vi "make_cursor_text.vi"(4 "Track Eye":T3, 5 "Cursor Position":T4, 6 "Scale":T1, 7 "Cursor Text":T2={"Cursor Name"="Cursor0", "Font Size"=7, "Show Position"=TRUE, "Show Name"=TRUE, "Text Color"=0, "Back Color"=16754450, "Opacity"=0.5}, 9 "Point Size":dbl, 10 "Cursor Name":string, 11 "Scene Cursor Object In":refnum<vi>) -> (3 "Scene Cursor Object Out":refnum<vi>)   [LabVIEW 2020, in "3DPC_SurfacePlot.xctl"]
uses:
  <vilib>/Native 3D Graph/xcontrol/3DPC_SurfacePlot.xctl
  <vilib>/Native 3D Graph/typedefs/prop_cursor_position.ctl
  <vilib>/Native 3D Graph/typedefs/track_eye.ctl
  <vilib>/Native 3D Graph/typedefs/vector.ctl
  <vilib>/Native 3D Graph/typedefs/prop_cursor_text.ctl
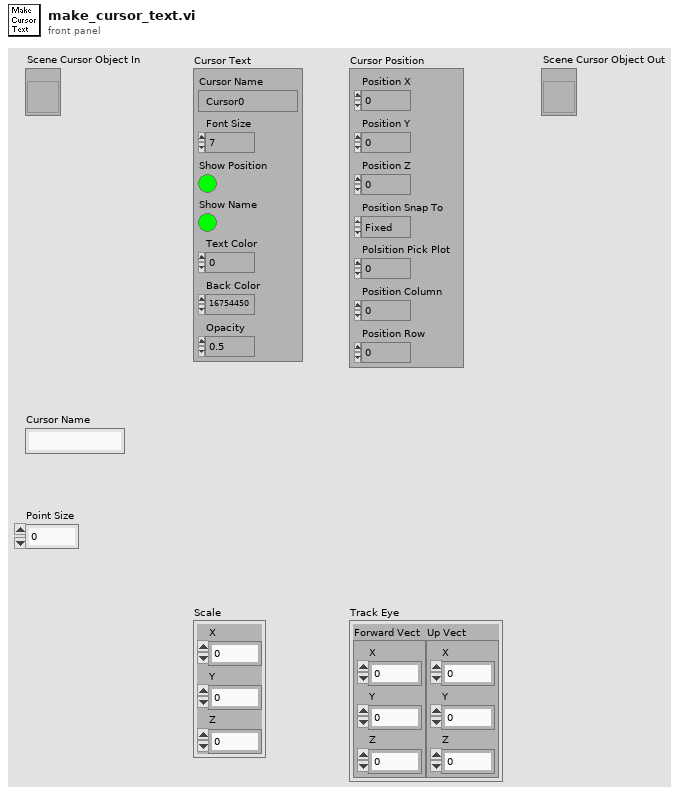
[diagram p1: front panel]
types:
  T1 = typedef "3DPC_SurfacePlot.xctl/vector.ctl" = cluster{"X":sgl, "Y":sgl, "Z":sgl}
  T2 = typedef "3DPC_SurfacePlot.xctl/prop_cursor_text.ctl" = cluster{"Cursor Name":string, "Font Size":i32, "Show Position":bool, "Show Name":bool, "Text Color":u32, "Back Color":u32, "Opacity":dbl}
  T3 = typedef "3DPC_SurfacePlot.xctl/track_eye.ctl" = cluster{"Forward Vect":T1, "Up Vect":T1}
  T4 = typedef "3DPC_SurfacePlot.xctl/prop_cursor_position.ctl" = cluster{"Position X":dbl, "Position Y":dbl, "Position Z":dbl, "Position Snap To":enum16{"Fixed", "Nearest Plot", "Snap to Plot"}, "Polsition Pick Plot":u16, "Position Column":i32, "Position Row":i32}
  T5 = enum8{"X-Y", "Y-Z", "X-Z", "Reversed X-Y", "Reversed Y-Z", "Reversed X-Z", "Screen"}
  T6 = enum16{"Normal Bin", "Opaque Bin", "Transparent Bin"}
  T7 = cluster{"Position X":dbl, "Position Y":dbl, "Position Z":dbl}
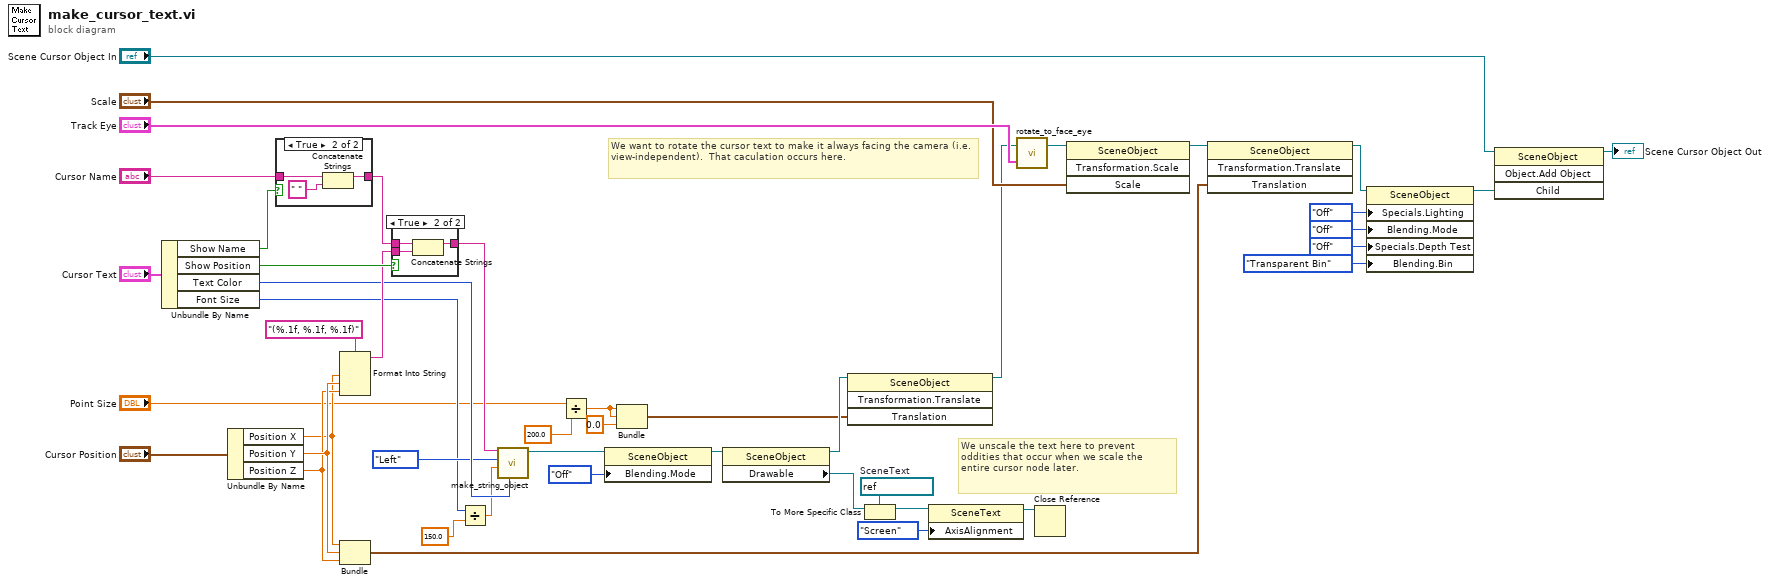
[diagram p0: block diagram]
diagram:
  w20 = refnum<vi> refnum  # SceneText
  # "We unscale the text here to prevent oddities that occur when we scale the entire cursor node later."
  # "We want to rotate the cursor text to make it always facing the camera (i.e. view-independent).  That caculation occurs here."
  n1 = Unbundle By Name("Cursor Text") -> ("Show Name"=w34:bool, "Show Position"=w33:bool, "Text Color"=w29:u32, "Font Size"=w12:i32)
  n2 = Unbundle By Name("Cursor Position") -> ("Position X"=w8:dbl, "Position Y"=w44:dbl, "Position Z"=w28:dbl)
  n3 = case shown="True" w34 {
    tunnel: "Cursor Name" -> [_ w48]
    tunnel: [_ w46] -> w32
    frame False {
    }
    frame True {
      n4 = Concatenate Strings(w48, " " ("string")) -> (w46:string)
    }
  }
  n5 = Format Into String(format string="(%.1f, %.1f, %.1f)", w8, w44, w28) -> (resulting string=w31:string)  [unwired: 2 in, 1 out]
  n6 = Bundle("Position X"=w8, "Position Y"=w44, "Position Z"=w28) -> (w42:T7)  [unwired: 1 out]
  n7 = case shown="True" w33 {
    tunnel: w32 -> [w49 w52]
    tunnel: w31 -> [_ w51]
    tunnel: [w49 w50] -> w30
    frame False {
    }
    frame True {
      n8 = Concatenate Strings(w52, w51) -> (w50:string)
    }
  }
  n9 = Divide(x=w12, y=150.0) -> (x/y=w9:dbl)
  n10 = call <vilib>:"make_string_object.vi"("Color"=w29, "Font Size"=w9, "Alignment:Horizontal"=enum8{"Left", "Right", "Center"}."Left", "String"=w30) -> ("String Object Out"=w26:refnum<vi>)  [unwired: 7 out]
  n11 = Divide(x="Point Size", y=200.0) -> (x/y=w3:dbl)
  n12 = property class="SceneObject"(reference=w26, "Blending.Mode"=enum16{"Inherit Value", "Off", "On"}."Off" ("Blending:Mode")) -> (reference out=w18:refnum<vi>)  [unwired: 1 in, 1 out]
  n13 = Bundle(w3, w3, "Z"=sgl 0.0) -> (w1:cluster{dbl, dbl, "Z":sgl})  [unwired: 1 out]
  n14 = property class="SceneObject"(reference=w18) -> (reference out=w7:refnum<vi>, "Drawable"=w17:refnum<vi>)  [unwired: 1 in, 1 out]
  n15 = invoke class="SceneObject" method="Transformation.Translate"(reference=w7, "Translation"=w1) -> (reference out=w6:refnum<vi>)  [unwired: 2 in, 3 out]
  n16 = To More Specific Class(target class=w20, reference=w17) -> (specific class reference=w16:refnum<vi>)  [unwired: 1 in, 1 out]
  n17 = property class="SceneText"(reference=w16, "AxisAlignment"=T5."Screen") -> (reference out=w15:refnum<vi>)  [unwired: 1 in, 1 out]
  n18 = call <vilib>:"rotate_to_face_eye.vi"("Track Eye"="Track Eye", "Object To Rotate"=w6) -> ("Rotated Object"=w10:refnum<vi>)  [unwired: 1 out]
  n19 = Close Reference(reference=w15) -> ()  [unwired: 1 in, 1 out]
  n20 = invoke class="SceneObject" method="Transformation.Scale"(reference=w10, "Scale"="Scale") -> (reference out=w14:refnum<vi>)  [unwired: 2 in, 3 out]
  n21 = invoke class="SceneObject" method="Transformation.Translate"(reference=w14, "Translation"=w42) -> (reference out=w24:refnum<vi>)  [unwired: 2 in, 3 out]
  n22 = property class="SceneObject"(reference=w24, "Specials.Lighting"=enum16{"Inherit Value", "Off", "On"}."Off" ("Specials:Lighting"), "Blending.Mode"=enum16{"Inherit Value", "Off", "On"}."Off" ("Blending:Mode"), "Specials.Depth Test"=enum16{"Inherit Value", "Off", "On"}."Off" ("Specials:Depth Test"), "Blending.Bin"=T6."Transparent Bin" ("Blending:Bin")) -> (reference out=w23:refnum<vi>)  [unwired: 1 in, 1 out]
  n23 = invoke class="SceneObject" method="Object.Add Object"(reference="Scene Cursor Object In", "Child"=w23) -> (reference out=→"Scene Cursor Object Out":refnum<vi>)  [unwired: 2 in, 3 out]
